vi "Set Target IP.vi"(8 "error in (no error)":errorcluster, 10 "IP":string, 11 "system definition in":refnum<k24>) -> (0 "error out":errorcluster, 3 "system definition out":refnum<k24>)   [LabVIEW 2013, in "Project Wizard.lvlib"]
uses:
  Project Wizard.lvlib
  NationalInstruments.VeriStand.SystemDefinitionAPI
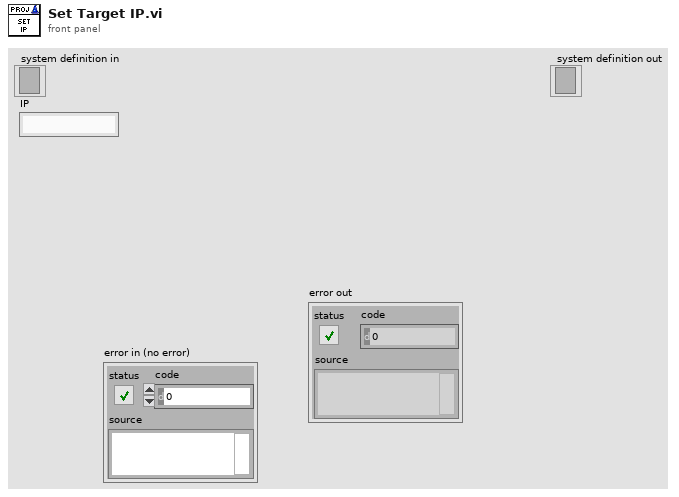
[diagram p1: front panel]
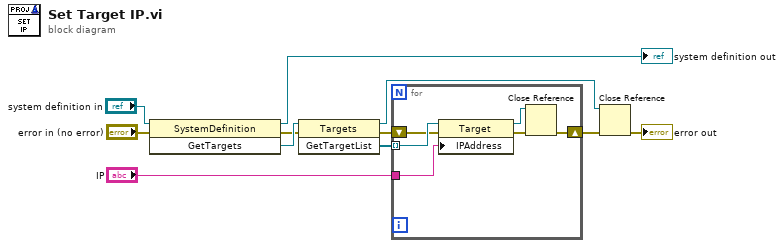
[diagram p0: block diagram]
diagram:
  n1 = invoke class="SystemDefinition" method="GetTargets"(reference="system definition in", error in="error in (no error)") -> (reference out=→"system definition out":refnum<k24>, error out=w4:errorcluster, "GetTargets"=w10:refnum<k24>)  [unwired: 1 in]
  n2 = invoke class="Targets" method="GetTargetList"(reference=w10, error in=w4) -> (reference out=w5:refnum<k24>, error out=w8:errorcluster, "GetTargetList"=w9:refnum<k24>[])  [unwired: 1 in]
  n3 = for {
    tunnel: w9 -> [w17] mode=indexing
    shift-right: [w12] -> w6
    shift-left: w8 -> [w16]
    tunnel: "IP" -> [w15]
    n4 = property class="Target"(reference=w17, error in=w16, "IPAddress"=w15) -> (reference out=w13:refnum<k24>, error out=w14:errorcluster)
    n5 = Close Reference(reference=w13, error in (no error)=w14) -> (error out=w12:errorcluster)
  }
  n6 = Close Reference(reference=w5, error in (no error)=w6) -> (error out=→"error out":errorcluster)
